vi "ScriptedAuto.vi"() -> ()   [LabVIEW 2013]
uses:
  AutoDriveParams.ctl
  Robot Global Data.vi
  Drivetrain/Drivetrain Set.vi
panel:
  out "Drive Params":T1
  out "Drive PID":T2={"X Dist"={"PID gains"={"proportional gain (Kc)"=1.0, "integral time (Ti, min)"=0.0, "derivative time (Td, min)"=0.0}, "output range"={"output high"=1.0, "output low"=-1.0}}, "Y Dist"={"PID gains"={"proportional gain (Kc)"=1.0, "integral time (Ti, min)"=0.0, "derivative time (Td, min)"=0.0}, "output range"={"output high"=1.0, "output low"=-1.0}}} {"Y Dist"."output range"."output low" format="%.2f"; "Y Dist"."output range"."output high" format="%.2f"; "Y Dist"."PID gains"."derivative time (Td, min)" format="%.3f"; "Y Dist"."PID gains"."integral time (Ti, min)" format="%.3f"; "Y Dist"."PID gains"."proportional gain (Kc)" format="%.3f"; "X Dist"."output range"."output low" format="%.2f"; "X Dist"."output range"."output high" format="%.2f"; "X Dist"."PID gains"."derivative time (Td, min)" format="%.3f"; "X Dist"."PID gains"."integral time (Ti, min)" format="%.3f"; "X Dist"."PID gains"."proportional gain (Kc)" format="%.3f"}
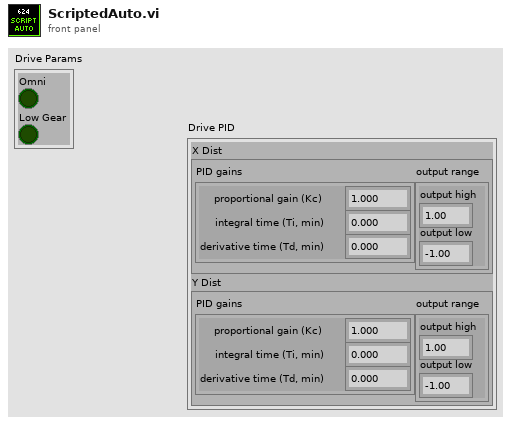
[diagram p1: front panel]
types:
  T1 = typedef "AutoDriveParams.ctl" = cluster{"Omni":bool, "Low Gear":bool}
  T2 = cluster{"X Dist":cluster{"PID gains":cluster{"proportional gain (Kc)":dbl, "integral time (Ti, min)":dbl, "derivative time (Td, min)":dbl}, "output range":cluster{"output high":dbl, "output low":dbl}}, "Y Dist":cluster{"PID gains":cluster{"proportional gain (Kc)":dbl, "integral time (Ti, min)":dbl, "derivative time (Td, min)":dbl}, "output range":cluster{"output high":dbl, "output low":dbl}}}
  T3 = typedef "Dashboard UDP Packet.ctl" = cluster{"Camera":T4, "Gyro":T5, "Encoder":T7, "Auto Shift":T8, "Auton":T9, "Drive/Ramp X":dbl, "Drive/Ramp Y":dbl, "Drive/Battery Cutoff":dbl, "Pressure/Compressor Min Voltage":dbl, "Pressure/Compressor Delay":dbl, "Controller/Strafe Correction":bool, "Shooter":T10, "Rollers":T11, "Abort":bool, "Finish":bool, "IR Halo Sustain Time":dbl, "Disable Compressor":bool, "Center Omni Drive Delay":i32, "Vision Mode":T12, "Radius Throttle":bool, "Fieldcentric":T13, "Roll":T14, "Stick Deadband":dbl}
  T4 = typedef "Camera Controls.ctl" = cluster{"Camera/View Angle X":dbl, "Camera/Goal Track Timeout":dbl, "Camera/View Angle Y":dbl, "Camera/Goal Exposure":dbl, "Camera/Vision Receive Timeout":dbl, "Camera/Offset 1":dbl, "Camera/Offset 2":dbl}
  T5 = typedef "Gyro Controls.ctl" = cluster{"Gyro/Angle Tolerance":dbl, "Gyro/Steer Closeness Threshold":dbl, "Steer PID":T6, "Steer Close PID":T6}
  T6 = typedef "PID Params.ctl" = cluster{"max":dbl, "min":dbl, "P":dbl, "I":dbl, "D":dbl}
  T7 = typedef "Encoder Controls.ctl" = cluster{"Encoders/Reset":bool, "Encoders/Omni Constant":dbl, "Encoders/Omni Tick Constant":dbl, "Encoders/Left Constant":dbl, "Encoders/Right Constant":dbl, "Encoders/Right Tick Constant":dbl}
  T8 = typedef "Auto Shift Controls.ctl" = cluster{"AutoShift/Upshift Throttle Accel":dbl, "AutoShift/Speed Threshold":dbl, "AutoShift/Upshift Throttle":dbl, "AutoShift/Upshift Accel":dbl, "AutoShift/Downshift Accel":dbl, "AutoShift/Downshift Throttle":dbl, "AutoShift/Delay":dbl, "AutoShift/Enabled":bool}
  T9 = typedef "Auton Controls.ctl" = cluster{"Auton/Left Shoot X-Coord":dbl, "Auton/Right Shoot X-Coord":dbl, "DistDrive/Distance Stop Threshold":dbl, "DistDrive/Max Stop Speed":dbl, "Auton/Back Piston Time":dbl, "Auton/Manual Hot":bool, "Auton/Manual Hot Right":bool, "Default X PID":T6, "Default Y PID":T6}
  T10 = typedef "Shooter Controls.ctl" = cluster{"Shooter/Reset Time":dbl, "Shooter/Release Delay":dbl, "Shooter/Pressure Steady Time":dbl, "Shooter/Misfire Delay":dbl, "Shooter/Ball Settle Time":dbl, "Shooter/Line IR Delay":dbl, "Pressure/Upper PSI Time":dbl, "Pressure/Lower PSI Time":dbl, "Shooter/Punch Delay":dbl, "Shooter/Target Pressure":dbl, "Pressure/Line B":dbl, "Pressure/Line M":dbl, "Pressure/Shooter M":dbl, "Pressure/Shooter B":dbl, "Halo Time":dbl, "Soft Release Delay":dbl, "Soft Unpin Delay":dbl, "Soft Shoot Delay":dbl}
  T11 = typedef "Roller Controls.ctl" = cluster{"Roller/Load IRs Verify Time":dbl, "Roller/Center IR Latch Time":dbl, "Roller/Speed Front":dbl, "Roller/Speed Back":dbl, "Roller/Entry Timeout":dbl, "Roller/To Center Timeout":dbl, "Roller/Sustain Time":dbl, "Roller/Verify Center Time":dbl}
  T12 = typedef "Vision Mode.ctl" = enum16{"Normal", "Extreme Left", "Extreme Right"}
  T13 = typedef "Fieldcentric Controls.ctl" = cluster{"Relative Angle":bool, "Point Robot":bool, "X/Y ratio low":dbl, "Steering Gain":dbl, "Force Omni Down":bool, "Enable":bool, "X/Y ratio high":dbl}
  T14 = typedef "Roll Maneuver.ctl" = cluster{"X 1":dbl, "Y 1":dbl, "Y 2":dbl, "X 2":dbl, "Y 3":dbl, "X 3":dbl, "Time 1":i32, "Time 2":i32, "Time 3":i32, "Angle Start":dbl, "Angle End":dbl, "Angle Linearity":dbl}
  T15 = cluster{"Gains":cluster{"P":dbl, "I":dbl, "D":dbl}, "Output Range":cluster{"max":dbl, "min":dbl}}
  T16 = cluster{"proportional gain (Kc)":dbl, "integral time (Ti, min)":dbl, "derivative time (Td, min)":dbl}
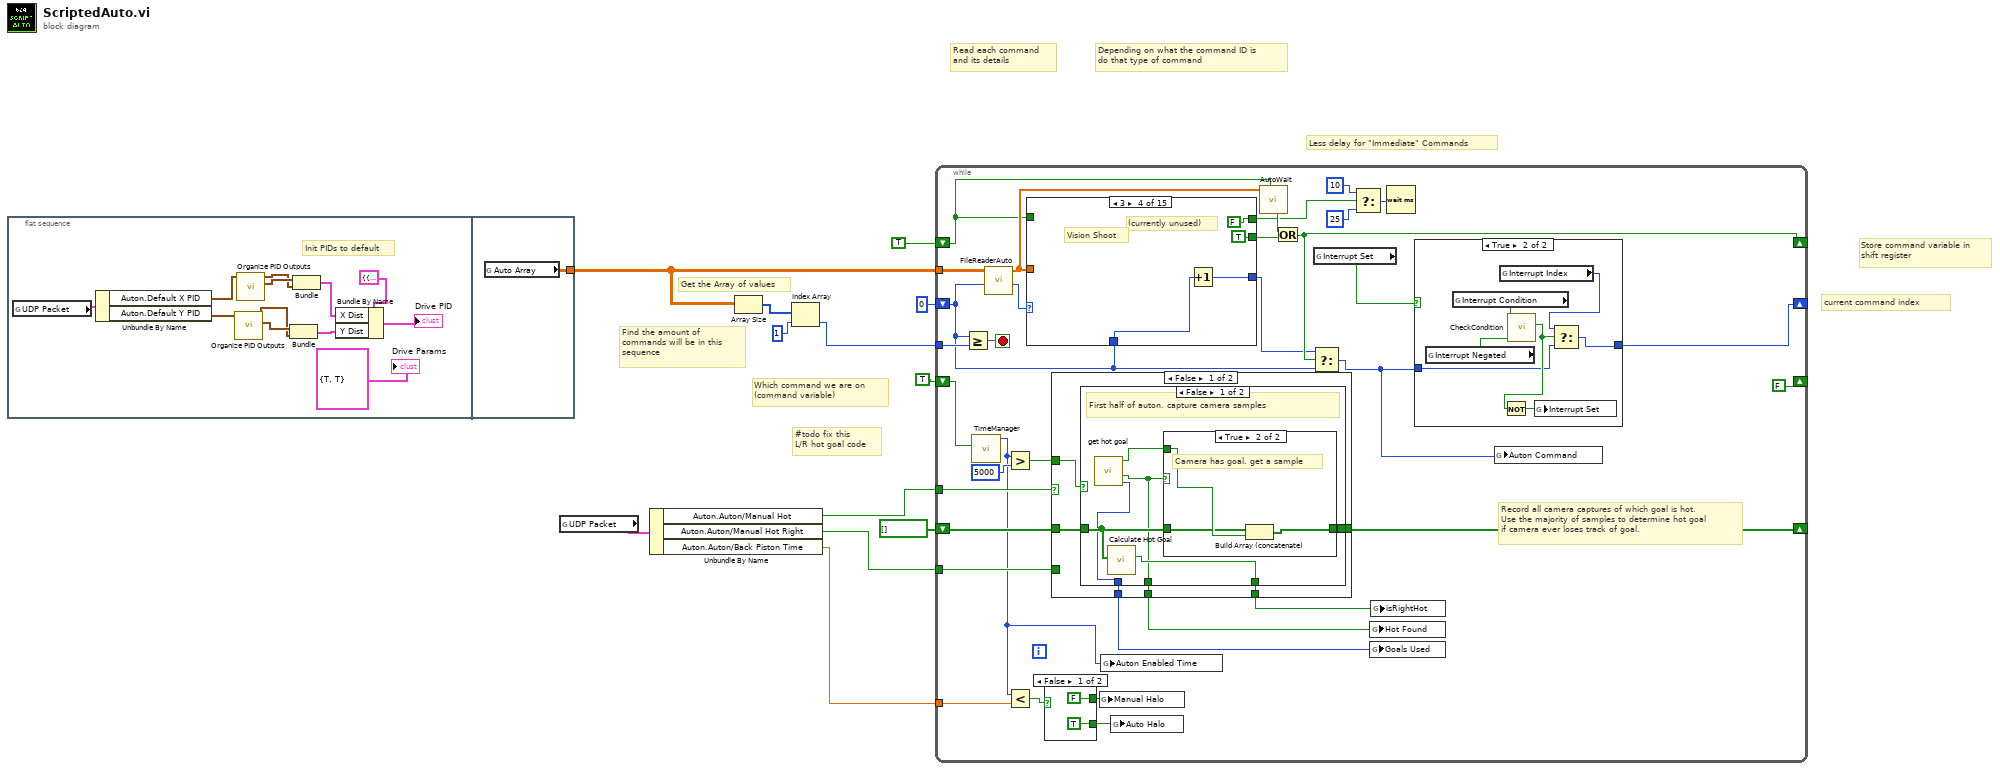
[diagram p0: block diagram]
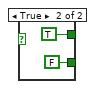
[diagram p2: hidden frame]
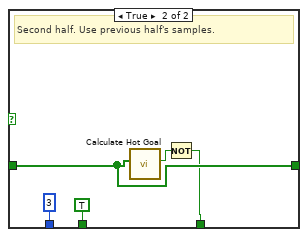
[diagram p4: hidden frame]
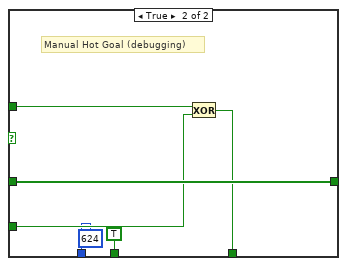
[diagram p5: hidden frame]
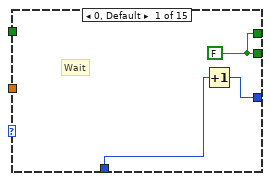
[diagram p7: hidden frame]
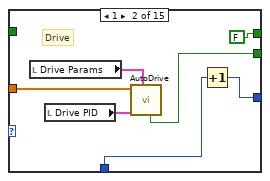
[diagram p8: hidden frame]
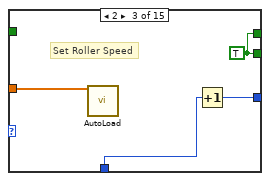
[diagram p9: hidden frame]
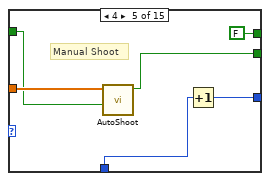
[diagram p10: hidden frame]
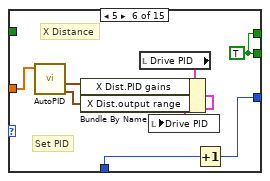
[diagram p11: hidden frame]
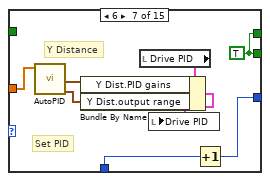
[diagram p12: hidden frame]
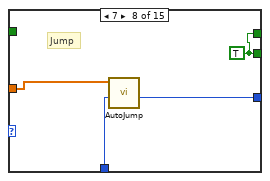
[diagram p13: hidden frame]
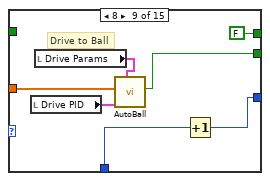
[diagram p14: hidden frame]
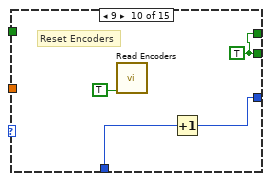
[diagram p15: hidden frame]
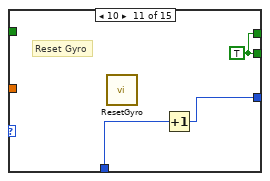
[diagram p16: hidden frame]
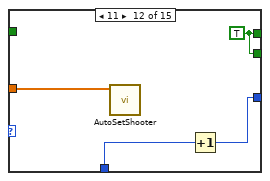
[diagram p17: hidden frame]
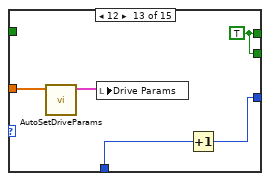
[diagram p18: hidden frame]
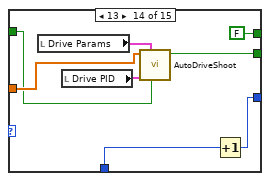
[diagram p19: hidden frame]
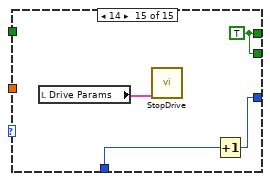
[diagram p20: hidden frame]
diagram:
  # "Less delay for \"Immediate\" Commands"
  # "current command index"
  # "Read each command\nand its details"
  # "#todo fix this\nL/R hot goal code"
  # "Which command we are on\n(command variable)"
  # "Store command variable in\nshift register"
  # "Depending on what the command ID is\ndo that type of command"
  # "Get the Array of values"
  # "Find the amount of \ncommands will be in this \nsequence"
  n1 = flat-sequence {
    tunnel: [w25] -> w6
    frame #0 {
      # "Init PIDs to default"
      n2 = global read "Robot Global Data.vi" "UDP Packet"() -> (w21:T3)
      n3 = Unbundle By Name(w21) -> ("Auton.Default X PID"=w20:T6, "Auton.Default Y PID"=w17:T6)
      n4 = call "Organize PID Outputs.vi"("PID"=w17) -> ("Gains"=w16:cluster{"P":dbl, "I":dbl, "D":dbl}, "Output Range"=w15:cluster{"max":dbl, "min":dbl})  [unwired: 9 in]
      n5 = call "Organize PID Outputs.vi"("PID"=w20) -> ("Gains"=w19:cluster{"P":dbl, "I":dbl, "D":dbl}, "Output Range"=w18:cluster{"max":dbl, "min":dbl})  [unwired: 9 in]
      n6 = Bundle("Gains"=w16, "Output Range"=w15) -> (w14:T15)  [unwired: 1 in]
      n7 = Bundle("Gains"=w19, "Output Range"=w18) -> (w13:T15)  [unwired: 1 in]
      n8 = Bundle By Name(cluster=T2 {"X Dist"={"PID gains"={"proportional gain (Kc)"=1.0, "integral time (Ti, min)"=0.0, "derivative time (Td, min)"=0.0}, "output range"={"output high"=0.93, "output low"=-0.93}}, "Y Dist"={"PID gains"={"proportional gain (Kc)"=1.0, "integral time (Ti, min)"=0.0, "derivative time (Td, min)"=0.0}, "output range"={"output high"=1.0, "output low"=-1.0}}} ("Drive PID"), "X Dist"=w13, "Y Dist"=w14) -> (→"Drive PID":T2)
      "Drive Params" <- T1 {"Omni"=TRUE, "Low Gear"=TRUE} ("Drive Params")
    }
    frame #1 {
      n9 = global read "Robot Global Data.vi" "Auto Array"() -> (w25:dbl[][])
    }
  }
  n10 = global read "Robot Global Data.vi" "UDP Packet"() -> (w4:T3)
  n11 = Unbundle By Name(w4) -> ("Auton.Auton/Manual Hot"=w3:bool, "Auton.Auton/Manual Hot Right"=w2:bool, "Auton.Auton/Back Piston Time"=w1:dbl)
  n12 = Array Size(array=w6) -> (size(s)=w12:i32[])
  n13 = Index Array(array=w12, index=1) -> (element=w11:i32)
  n14 = while {
    tunnel: w6 -> [w52]
    tunnel: w11 -> [w59]
    shift-right: [w49] -> _
    shift-left: 0 -> [w43]
    shift-right: [w44] -> _
    shift-left: TRUE -> [w45]
    shift-right: [FALSE] -> _
    shift-left: TRUE -> [w50]
    shift-right: [w47] -> _
    shift-left: bool[] [] -> [w48]
    tunnel: w3 -> [w35]
    tunnel: w2 -> [w34]
    tunnel: w1 -> [w29]
    stop <- w58 stop-if-true
    # "Record all camera captures of which goal is hot.\nUse the majority of samples to determine hot goal\nif camera ever loses track of goal."
    n15 = Greater Or Equal?(x=w43, y=w59) -> (x >= y?=w58:bool)
    n16 = call "TimeManager.vi"("Reset?"=w50) -> ("Time Since Reset"=w26:u32)  [unwired: 9 in, 1 out]
    n17 = call "FileReaderAuto.vi"("index"=w43, "Auto Array"=w52) -> ("Command ID"=w54:i16, "Array"=w53:dbl[])  [unwired: 8 in]
    n18 = Greater?(x=w26, y=u32 5000) -> (0:w46:bool)
    n19 = Less?(x=w26, y=w29) -> (x < y?=w27:bool)
    n20 = case shown="3" w54 {
      tunnel: w53 -> [_ w106 w110 _ w119 w126 w134 w142 w147 _ _ w160 w164 w168 _]
      tunnel: [w99 w105 w109 TRUE ("isFinished") w120 w123 w131 w139 w145 w150 w154 w159 w163 w166 w175] -> w57
      tunnel: w45 -> [_ _ _ _ w118 _ _ _ _ _ _ _ _ w167 _]
      tunnel: w43 -> [w100 w107 w111 w115 w121 w130 w138 w141 w148 w152 w156 w158 w161 w172 w177]
      tunnel: [w101 w108 w112 w116 w122 w129 w137 w140 w149 w151 w155 w157 w162 w171 w176] -> w41
      tunnel: [w99 FALSE ("isFinished") w109 FALSE ("isFinished") FALSE ("isFinished") w123 w131 w139 FALSE ("isFinished") w150 w154 w159 w163 FALSE ("isFinished") w175] -> w37
      frame 0, Default {
        w99 = FALSE
        # "Wait"
        n21 = Increment(x=w100) -> (x+1=w101:i32)
      }
      frame 1 {
        # "Drive"
        n22 = local read "Drive Params"() -> (w102:T1)
        n23 = local read "Drive PID"() -> (w104:T2)
        n24 = call "AutoDrive.vi"("Drive Params"=w102, "Drive PID"=w104, "Array"=w106) -> ("isFinished"=w105:bool)  [unwired: 8 in]
        n25 = Increment(x=w107) -> (x+1=w108:i32)
      }
      frame 2 {
        w109 = TRUE ("isFinished")
        # "Set Roller Speed"
        n26 = call "AutoLoad.vi"("Array"=w110) -> ()  [unwired: 11 in]
        n27 = Increment(x=w111) -> (x+1=w112:i32)
      }
      frame 3 {
        # "(currently unused)"
        # "Vision Shoot"
        n28 = Increment(x=w115) -> (x+1=w116:i32)
      }
      frame 4 {
        # "Manual Shoot"
        n29 = call "AutoShoot.vi"("Reset?"=w118, "Array"=w119) -> ("isFinished"=w120:bool)  [unwired: 9 in]
        n30 = Increment(x=w121) -> (x+1=w122:i32)
      }
      frame 5 {
        w123 = TRUE ("isFinished")
        # "X Distance"
        # "Set PID"
        n31 = call "AutoPID.vi"("Array"=w126) -> ("output range"=w128:cluster{"output high":dbl, "output low":dbl}, "PID gains"=w127:T16)  [unwired: 9 in]
        n32 = local read "Drive PID"() -> (w125:T2)
        n33 = Bundle By Name(cluster=w125, "X Dist.PID gains"=w127, "X Dist.output range"=w128) -> (w124:T2)
        n34 = local write "Drive PID"(w124) -> ()
        n35 = Increment(x=w130) -> (x+1=w129:i32)
      }
      frame 6 {
        w131 = TRUE ("isFinished")
        # "Y Distance"
        # "Set PID"
        n36 = call "AutoPID.vi"("Array"=w134) -> ("output range"=w136:cluster{"output high":dbl, "output low":dbl}, "PID gains"=w135:T16)  [unwired: 9 in]
        n37 = local read "Drive PID"() -> (w133:T2)
        n38 = Bundle By Name(cluster=w133, "Y Dist.PID gains"=w135, "Y Dist.output range"=w136) -> (w132:T2)
        n39 = local write "Drive PID"(w132) -> ()
        n40 = Increment(x=w138) -> (x+1=w137:i32)
      }
      frame 7 {
        w139 = TRUE ("isFinished")
        # "Jump"
        n41 = call "AutoJump.vi"("Current Index"=w141, "Array"=w142) -> ("New Index"=w140:i32)  [unwired: 9 in]
      }
      frame 8 {
        # "Drive to Ball"
        n42 = local read "Drive PID"() -> (w146:T2)
        n43 = local read "Drive Params"() -> (w143:T1)
        n44 = call "AutoBall.vi"("Drive Params"=w143, "PID Params"=w146, "Command Array"=w147) -> ("isFinished"=w145:bool)  [unwired: 8 in]
        n45 = Increment(x=w148) -> (x+1=w149:i32)
      }
      frame 9 {
        w150 = TRUE ("isFinished")
        # "Reset Encoders"
        n46 = call "Read Encoders.vi"("Reset"=TRUE) -> ()  [unwired: 10 in, 1 out]
        n47 = Increment(x=w152) -> (x+1=w151:i32)
      }
      frame 10 {
        w154 = TRUE ("isFinished")
        # "Reset Gyro"
        n48 = call "ResetGyro.vi"() -> ()  [unwired: 12 in]
        n49 = Increment(x=w156) -> (x+1=w155:i32)
      }
      frame 11 {
        w159 = TRUE ("isFinished")
        n50 = call "AutoSetShooter.vi"("Array"=w160) -> ()  [unwired: 11 in]
        n51 = Increment(x=w158) -> (x+1=w157:i32)
      }
      frame 12 {
        w163 = TRUE ("isFinished")
        n52 = call "AutoSetDriveParams.vi"("Array"=w164) -> ("Drive Params"=w165:cluster{"Omni":bool, "Low Gear":bool})  [unwired: 10 in]
        n53 = local write "Drive Params"(w165) -> ()
        n54 = Increment(x=w161) -> (x+1=w162:i32)
      }
      frame 13 {
        n55 = local read "Drive Params"() -> (w170:T1)
        n56 = local read "Drive PID"() -> (w169:T2)
        n57 = call "AutoDriveShoot.vi"("Reset?"=w167, "Drive Params"=w170, "Drive PID"=w169, "Array"=w168) -> ("Finished"=w166:bool)  [unwired: 7 in]
        n58 = Increment(x=w172) -> (x+1=w171:i32)
      }
      frame 14 {
        w175 = TRUE ("isFinished")
        n59 = local read "Drive Params"() -> (w174:T1)
        n60 = call "StopDrive.vi"("Drive Params"=w174) -> ()  [unwired: 11 in]
        n61 = Increment(x=w177) -> (x+1=w176:i32)
      }
    }
    n62 = case shown="False" w27 {
      tunnel: [TRUE ("Manual Halo") FALSE ("Manual Halo")] -> w30
      tunnel: [FALSE ("Manual Halo") TRUE ("Manual Halo")] -> w28
      frame False {
      }
      frame True {
      }
    }
    n63 = case shown="False" w35 {
      tunnel: w48 -> [w69 w90]
      tunnel: [w68 w90] -> w47
      tunnel: w46 -> [w67 w89]
      tunnel: [w66 w88] -> w36
      tunnel: w34 -> [_ w87]
      tunnel: [w65 TRUE ("Hot Goal Found")] -> w33
      tunnel: [w64 624] -> w32
      frame False {
        n64 = case shown="False" w67 {
          tunnel: w69 -> [w74 w84]
          tunnel: [w75 w84] -> w68
          tunnel: [w73 w82] -> w66
          tunnel: [w71 TRUE ("Hot Goal Found")] -> w65
          tunnel: [w70 3 ("Goals Used")] -> w64
          frame False {
            # "First half of auton. capture camera samples"
            n65 = call "get hot goal.vi"() -> ("Goals Used"=w70:i32, "Hot Goal Found"=w71:bool, "Right Hot"=w72:bool)  [unwired: 9 in]
            n66 = call "Calculate Hot Goal.vi"("Camera Samples"=w74) -> ("Right Hot?"=w73:bool)  [unwired: 9 in, 1 out]
            n67 = case shown="True" w71 {
              tunnel: w72 -> [_ w79]
              tunnel: w74 -> [w76 w78]
              tunnel: [w76 w77] -> w75
              frame False {
                # "Goal not found. Leave\nsample array unchanged"
              }
              frame True {
                # "Camera has goal. get a sample"
                n68 = Build Array (concatenate)(w78, w79) -> (w77:bool[])
              }
            }
          }
          frame True {
            # "Second half. Use previous half's samples."
            n69 = call "Calculate Hot Goal.vi"("Camera Samples"=w84) -> ("Right Hot?"=w83:bool)  [unwired: 9 in, 1 out]
            n70 = Not(x=w83) -> (.not. x?=w82:bool)
          }
        }
      }
      frame True {
        # "Manual Hot Goal (debugging)"
        n71 = Exclusive Or(1:w87, 2:w89) -> (0:w88:bool)
      }
    }
    n72 = global write "Robot Global Data.vi" "Manual Halo"(w28) -> ()
    n73 = global write "Robot Global Data.vi" "Auton Enabled Time"(w26) -> ()
    n74 = global write "Robot Global Data.vi" "Auto Halo"(w30) -> ()
    n75 = call "AutoWait.vi"("Reset?"=w45, "Array"=w53) -> ("isFinished"=w51:bool)  [unwired: 9 in]
    n76 = Or(x=w51, y=w57) -> (x .or. y?=w44:bool)
    n77 = Select(t=w41, s=w44, f=w43) -> (s? t:f=w31:i32)
    n78 = global read "Robot Global Data.vi" "Interrupt Set"() -> (w42:bool)
    n79 = Select(t=u32 10 ("milliseconds to wait"), s=w37, f=u32 25 ("milliseconds to wait")) -> (s? t:f=w40:u32)
    n80 = global write "Robot Global Data.vi" "Hot Found"(w33) -> ()
    n81 = global write "Robot Global Data.vi" "Goals Used"(w32) -> ()
    n82 = global write "Robot Global Data.vi" "isRightHot"(w36) -> ()
    n83 = Wait (ms)(milliseconds to wait=w40) -> ()  [unwired: 1 out]
    n84 = case shown="True" w42 {
      tunnel: w31 -> [w91 w93]
      tunnel: [w91 w98] -> w49
      frame False {
      }
      frame True {
        n85 = global read "Robot Global Data.vi" "Interrupt Negated"() -> (w92:bool)
        n86 = global read "Robot Global Data.vi" "Interrupt Condition"() -> (w97:i32)
        n87 = global read "Robot Global Data.vi" "Interrupt Index"() -> (w96:i32)
        n88 = call "CheckCondition.vi"("Negate"=w92, "Condition"=w97) -> ("Condition True?"=w94:bool)  [unwired: 9 in]
        n89 = Not(x=w94) -> (.not. x?=w95:bool)
        n90 = global write "Robot Global Data.vi" "Interrupt Set"(w95) -> ()
        n91 = Select(t=w96, s=w94, f=w93) -> (s? t:f=w98:i32)
      }
    }
    n92 = global write "Robot Global Data.vi" "Auton Command"(w31) -> ()
  }
